vi "Data Update.vi"(8 "error in (no error)":errorcluster, 10 "Data to Send":string, 11 "Nested Actor in":refnum<class "Nested Actor.lvclass">) -> (0 "error out":errorcluster, 3 "Nested Actor out":refnum<class "Nested Actor.lvclass">)   [LabVIEW 2020, in "Nested Actor.lvlib" / "Nested Actor.lvclass"]
uses:
  Nested Actor.lvclass
  E:/Program Files (x86)/National Instruments/LabVIEW 2020/vi.lib/ActorFramework/Actor/Actor.lvclass
  <vilib>/ActorFramework/Actor/Actor.lvclass/Actor.ctl
  Send String Messages/Data Received Msg/Data Received Msg.lvclass/Data Received Msg.ctl
  <vilib>/ActorFramework/Message Enqueuer/Message Enqueuer.lvclass/Message Enqueuer.ctl
  <vilib>/ActorFramework/Message Enqueuer/Enqueue.vi
  Send String Messages/Data Received Msg/Data Received Msg.lvclass
  E:/Program Files (x86)/National Instruments/LabVIEW 2020/vi.lib/ActorFramework/Message/Message.lvclass
  <vilib>/ActorFramework/Message Priority Queue/Priority Enqueue.vi
  <vilib>/ActorFramework/Actor/Actor.lvclass
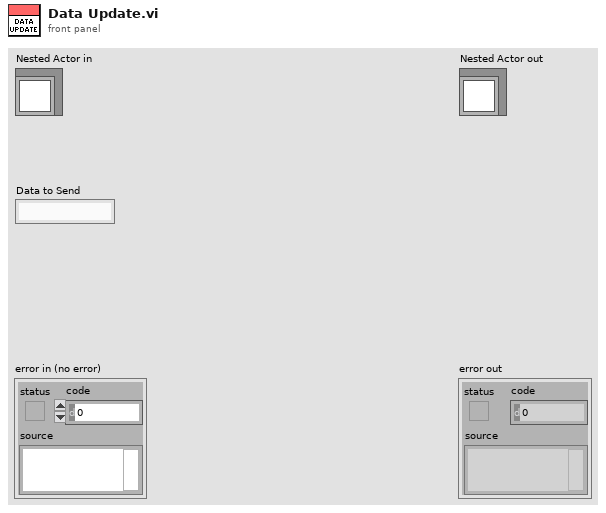
[diagram p1: front panel]
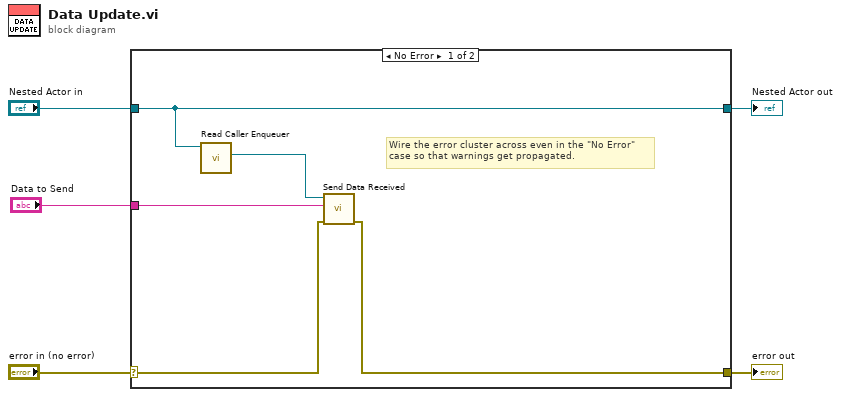
[diagram p0: block diagram]
diagram:
  n1 = case shown="No Error" "error in (no error)" {
    selector: "error in (no error)" -> [w7 w12]
    tunnel: [w6 w12] -> w4
    tunnel: [w10 w11] -> w2
    tunnel: "Nested Actor in" -> [w10 w11]
    tunnel: "Data to Send" -> [w8 _]
    frame No Error {
      # "Wire the error cluster across even in the \"No Error\"\ncase so that warnings get propagated."
      n2 = call <vilib>:"Read Caller Enqueuer.vi"("Actor"=w10) -> ("Caller Enqueuer"=w9:refnum<class "Message Enqueuer.lvclass">)  [unwired: 10 in]
      n3 = call "Send Data Received.vi"("error in (no error)"=w7, "Updated Data"=w8, "Message Enqueuer"=w9) -> ("error out"=w6:errorcluster)  [unwired: 7 in, 1 out]
    }
    frame Error {
    }
  }
  "error out" <- w4
  "Nested Actor out" <- w2
